vi "RTExampleQueryServer.vi"() -> ()   [LabVIEW 2019]
uses:
  VIs/QueryServer_AnalogInputData.ctl
  VIs/labview-grpc-query-server.lvlib
  VIs/gprc-support.lvlib
panel:
  in  "# of Measurements":i32=10
  in  "Server Key File (.key)":path
  in  "Server Certificate File (.crt)":path
  in  "stop":bool
  in  "Server Address":string="0.0.0.0:50051"
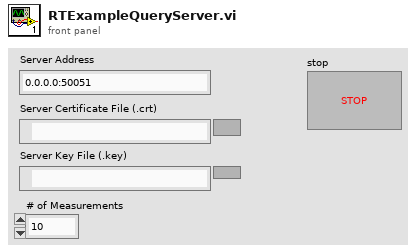
[diagram p1: front panel]
types:
  T1 = typedef "gprc-support.lvlib/grpcId.ctl" = u64
  T2 = cluster{"QueryServer_Invoke":refnum<user-event>, "QueryServer_Query":refnum<user-event>, "QueryServer_Register":refnum<user-event>, "QueryServer_TestDataTypes":refnum<user-event>, "QueryServer_PerformAnalogInput":refnum<user-event>, "gRPCid":T1}
  T3 = typedef "labview-grpc-query-server.lvlib/QueryServer_TestDataTypesParameters.ctl" = cluster{"Root":string, "Repeated String":string[], "Repeated Int32":i32[], "Root Int32":i32, "Root Bool":bool, "Repeated Double":dbl[], "Root Double":dbl, "Repeated Bool":bool[], "Root Float":sgl, "Repeated Float":sgl[], "DataTypeTest":T4, "Repeated Nested":T4[]}
  T4 = typedef "labview-grpc-query-server.lvlib/QueryServer_DataTypeTest.ctl" = cluster{"Bool Value":bool, "Int Value":i32, "Float Value":sgl, "Double Value":dbl}
  T5 = typedef "labview-grpc-query-server.lvlib/QueryServer_AnalogInputData.ctl" = cluster{"RepeatedDMMValue":sgl[], "RepeatedDAQValue0":sgl[], "RepeatedDAQValue1":sgl[], "RepeatedDAQValue2":sgl[], "RepeatedDAQValue3":sgl[], "RepeatedDAQValue4":sgl[], "RepeatedDAQValue5":sgl[], "RepeatedDAQValue6":sgl[], "RepeatedDAQValue7":sgl[], "t0":string, "dt":sgl, "errorstatus":bool, "errorcode":i32, "errorsource":string}
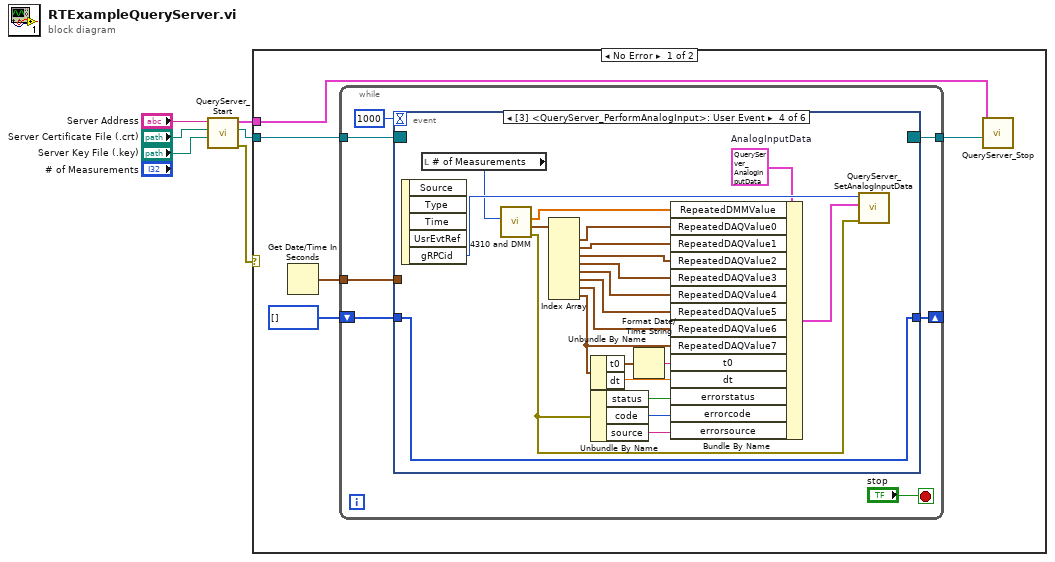
[diagram p0: block diagram]
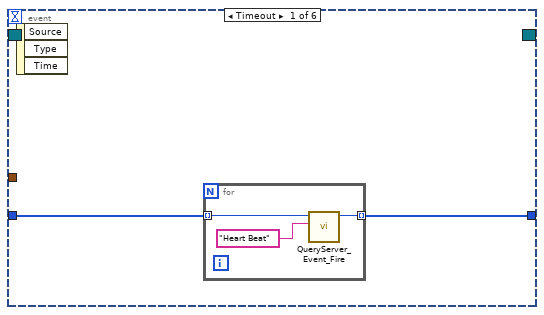
[diagram p2: hidden frame]
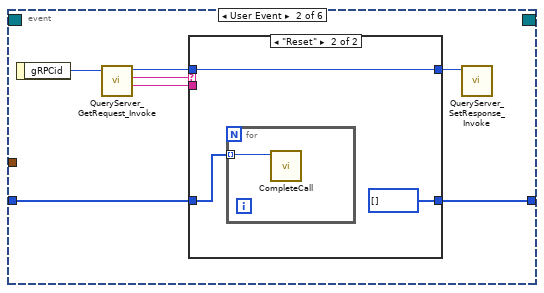
[diagram p3: hidden frame]
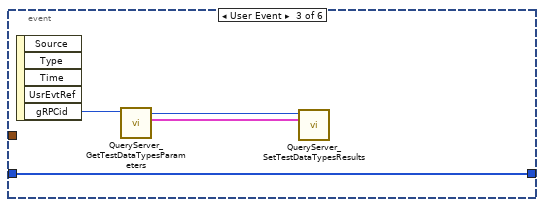
[diagram p5: hidden frame]
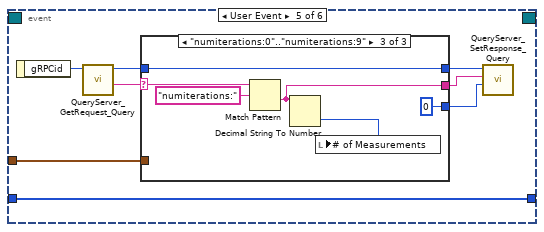
[diagram p6: hidden frame]
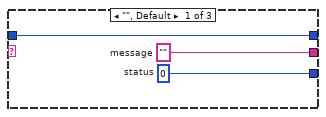
[diagram p7: hidden frame]
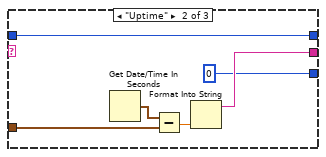
[diagram p8: hidden frame]
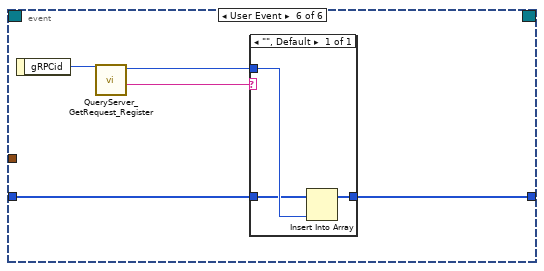
[diagram p9: hidden frame]
diagram:
  n1 = call "QueryServer_Start.vi"("Server Key File (.key)"="Server Key File (.key)", "Server Certificate File (.crt)"="Server Certificate File (.crt)", "Server Address"="Server Address") -> ("error out"=w2:errorcluster, "Event Registration Refnum"=w1:refnum<event-registration>, "Server Info"=w5:T2)  [unwired: 5 in]
  n2 = case shown="No Error" w2 {
    tunnel: w5 -> [w9 _]
    tunnel: w1 -> [w7 _]
    frame No Error {
      n3 = Get Date/Time In Seconds() -> (seconds since 1Jan1904=w11:timestamp)
      n4 = while {
        tunnel: [w17] -> w8
        tunnel: w11 -> [w16]
        shift-right: [w14] -> _
        shift-left: u64[] [] -> [w13]
        tunnel: w7 -> [w12]
        stop <- "stop" stop-if-true
        n5 = event shown="[3] <QueryServer_PerformAnalogInput>: User Event" {
          selector: w12 -> [_ _ _ _ _ _]
          dyn-events: [_ _ _ _ _ _] -> w17
          timeout: 1000 -> [_ _ _ _ _ _]
          tunnel: w16 -> [_ _ _ _ w65 _]
          tunnel: [w20 w24 w37 w50 w64 w88] -> w14
          tunnel: w13 -> [w19 w25 w37 w50 w64 w87]
          event Timeout {
            n6 = event-data() -> ()  [unwired: 1 in, 3 out]
            n7 = for {
              tunnel: w19 -> [w23] mode=indexing
              tunnel: [w21] -> w20 mode=indexing
              n8 = call "QueryServer_Event_Fire.vi"("eventdata"="Heart Beat", "gRPCid"=w23) -> ("gRPCid out"=w21:T1)  [unwired: 8 in, 1 out]
            }
          }
          event User Event {
            n9 = event-data() -> ("gRPCid"=w30:T1)  [unwired: 1 in]
            n10 = call "QueryServer_GetRequest_Invoke.vi"("gRPCid"=w30) -> ("parameter"=w26:string, "command"=w29:string, "gRPCid out"=w28:T1)  [unwired: 5 in, 1 out]
            n11 = case shown="\"Reset\"" w29 {
              tunnel: w28 -> [w32 w33]
              tunnel: [w32 w33] -> w27
              tunnel: w26 -> [_ _]
              tunnel: w25 -> [w31 w35]
              tunnel: [w31 u64[] []] -> w24
              frame "", Default {
              }
              frame "Reset" {
                n12 = for {
                  tunnel: w35 -> [w36] mode=indexing
                  n13 = call "CompleteCall.vi"("gRPCid"=w36) -> ()  [unwired: 9 in, 1 out]
                }
              }
            }
            n14 = call "QueryServer_SetResponse_Invoke.vi"("gRPCid"=w27) -> ()  [unwired: 9 in, 1 out]
          }
          event User Event {
            n15 = event-data() -> ("gRPCid"=w40:T1)  [unwired: 1 in, 4 out]
            n16 = call "QueryServer_GetTestDataTypesParameters.vi"("gRPCid"=w40) -> ("TestDataTypesParameters"=w39:T3, "gRPCid out"=w38:T1)  [unwired: 6 in, 1 out]
            n17 = call "QueryServer_SetTestDataTypesResults.vi"("TestDataTypesParameters"=w39, "gRPCid"=w38) -> ()  [unwired: 6 in, 2 out]
          }
          event User Event {
            w61 = T5 {"RepeatedDMMValue"=[], "RepeatedDAQValue0"=[], "RepeatedDAQValue1"=[], "RepeatedDAQValue2"=[], "RepeatedDAQValue3"=[], "RepeatedDAQValue4"=[], "RepeatedDAQValue5"=[], "RepeatedDAQValue6"=[], "RepeatedDAQValue7"=[], "t0"="", "dt"=0.0, "errorstatus"=FALSE, "errorcode"=0, "errorsource"=""}  # AnalogInputData
            n18 = event-data() -> ("gRPCid"=w62:T1)  [unwired: 1 in, 4 out]
            n19 = local read "# of Measurements"() -> (w41:i32)
            n20 = call "4310 and DMM.vi"("Number of Iterations"=w41) -> ("error out"=w45:errorcluster, "4309 Measurements"=w58:waveform(dbl)[], "DMM Measurements"=w60:dbl[])  [unwired: 8 in]
            n21 = Index Array(array=w58) -> (element #1=w57:waveform(dbl), element #2=w56:waveform(dbl), element #3=w55:waveform(dbl), element #4=w54:waveform(dbl), element #5=w53:waveform(dbl), element #6=w52:waveform(dbl), element #7=w51:waveform(dbl), element #8=w49:waveform(dbl))  [unwired: 8 in]
            n22 = Unbundle By Name(w49) -> ("t0"=w48:timestamp, "dt"=w46:dbl)
            n23 = Unbundle By Name(w45) -> ("status"=w44:bool, "code"=w43:i32, "source"=w42:string)
            n24 = Format Date/Time String(seconds (now)=w48) -> (date/time string=w47:string)  [unwired: 2 in]
            n25 = Bundle By Name(cluster=w61, "RepeatedDMMValue"=w60, "RepeatedDAQValue0"=w57, "RepeatedDAQValue1"=w56, "RepeatedDAQValue2"=w55, "RepeatedDAQValue3"=w54, "RepeatedDAQValue4"=w53, "RepeatedDAQValue5"=w52, "RepeatedDAQValue6"=w51, "RepeatedDAQValue7"=w49, "t0"=w47, "dt"=w46, "errorstatus"=w44, "errorcode"=w43, "errorsource"=w42) -> (w59:T5)
            n26 = call "QueryServer_SetAnalogInputData.vi"("error in (no error)"=w45, "AnalogInputData"=w59, "gRPCid"=w62) -> ()  [unwired: 5 in, 2 out]
          }
          event User Event {
            n27 = event-data() -> ("gRPCid"=w70:T1)  [unwired: 1 in]
            n28 = call "QueryServer_GetRequest_Query.vi"("gRPCid"=w70) -> ("gRPCid out"=w69:T1, "query"=w63:string)  [unwired: 7 in, 1 out]
            n29 = case shown="\"numiterations:0\"..\"numiterations:9\"" w63 {
              selector: w63 -> [_ _ w84]
              tunnel: w69 -> [w73 w75 w81]
              tunnel: [w73 w75 w81] -> w68
              tunnel: [w72 w76 w83] -> w67
              tunnel: [w71 0 ("status") 0 ("status")] -> w66
              tunnel: w65 -> [_ w78 _]
              frame "", Default {
                w71 = 0  # status
                w72 = ""  # message
              }
              frame "Uptime" {
                n30 = Get Date/Time In Seconds() -> (seconds since 1Jan1904=w79:timestamp)
                n31 = Subtract(x=w79, y=w78) -> (x-y=w77:dbl)
                n32 = Format Into String(w77) -> (resulting string=w76:string)  [unwired: 3 in, 1 out]
              }
              frame "numiterations:0".."numiterations:9" {
                n33 = Match Pattern(string=w84, regular expression="numiterations:") -> (after substring=w83:string)  [unwired: 1 in, 3 out]
                n34 = Decimal String To Number(string=w83) -> (number=w80:i32)  [unwired: 2 in, 1 out]
                n35 = local write "# of Measurements"(w80) -> ()
              }
            }
            n36 = call "QueryServer_SetResponse_Query.vi"("gRPCid"=w68, "message"=w67, "status"=w66) -> ()  [unwired: 7 in, 1 out]
          }
          event User Event {
            n37 = event-data() -> ("gRPCid"=w90:T1)  [unwired: 1 in]
            n38 = call "QueryServer_GetRequest_Register.vi"("gRPCid"=w90) -> ("gRPCid out"=w89:T1, "eventname"=w86:string)  [unwired: 7 in, 1 out]
            n39 = case shown="\"\", Default" w86 {
              tunnel: w89 -> [w93]
              tunnel: [w92] -> w88
              tunnel: w87 -> [w91]
              frame "", Default {
                n40 = Insert Into Array(array=w91, new element=w93) -> (w92:T1[])  [unwired: 1 in]
              }
            }
          }
        }
      }
      n41 = call "QueryServer_Stop.vi"("Server Info"=w9, "Event Registration Refnum"=w8) -> ()  [unwired: 8 in, 1 out]
    }
    frame Error {
    }
  }
